vi "Set2DPlots.vi"(2 "error in (no error)":errorcluster, 3 "ScanCoords [mm]":T1, 4 "Order selection":u16(ring)=1 items=["X->Z->Y"=6, "Y->Z->X"=5, "Z->X->Y"=3, "Y->X->Z"=2, "Z->Y->X"=4, "X->Y->Z"=1], 5 "2D graph 3":refnum<vi>) -> (0 "error out":errorcluster, 1 "initialized array":dbl[][](array[numeric]))   [LabVIEW 2015]
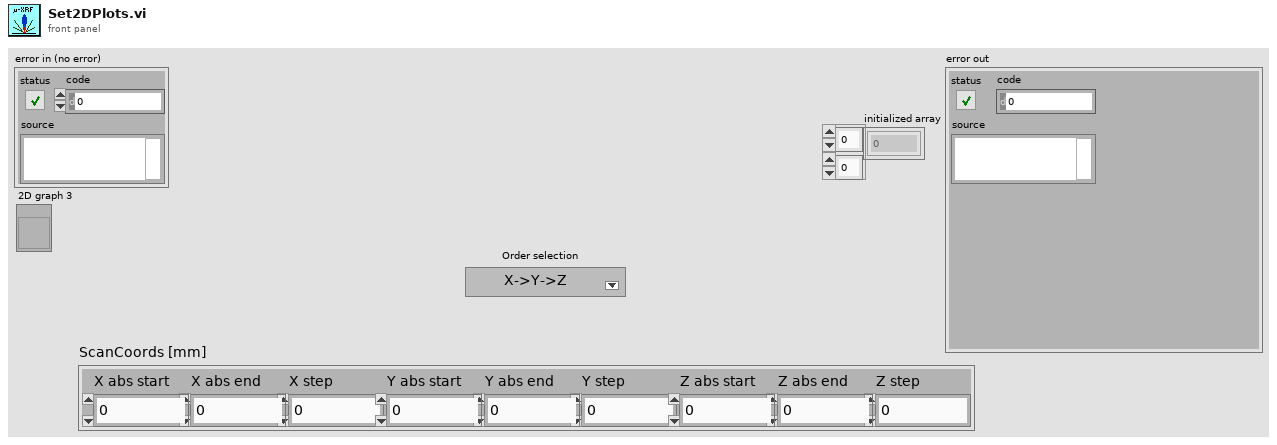
[diagram p1: front panel]
types:
  T1 = cluster{"X abs start":dbl, "X abs end":dbl, "Y abs start":dbl, "Y abs end":dbl, "Z abs start":dbl, "Z abs end":dbl, "X step":dbl, "Y step":dbl, "Z step":dbl}
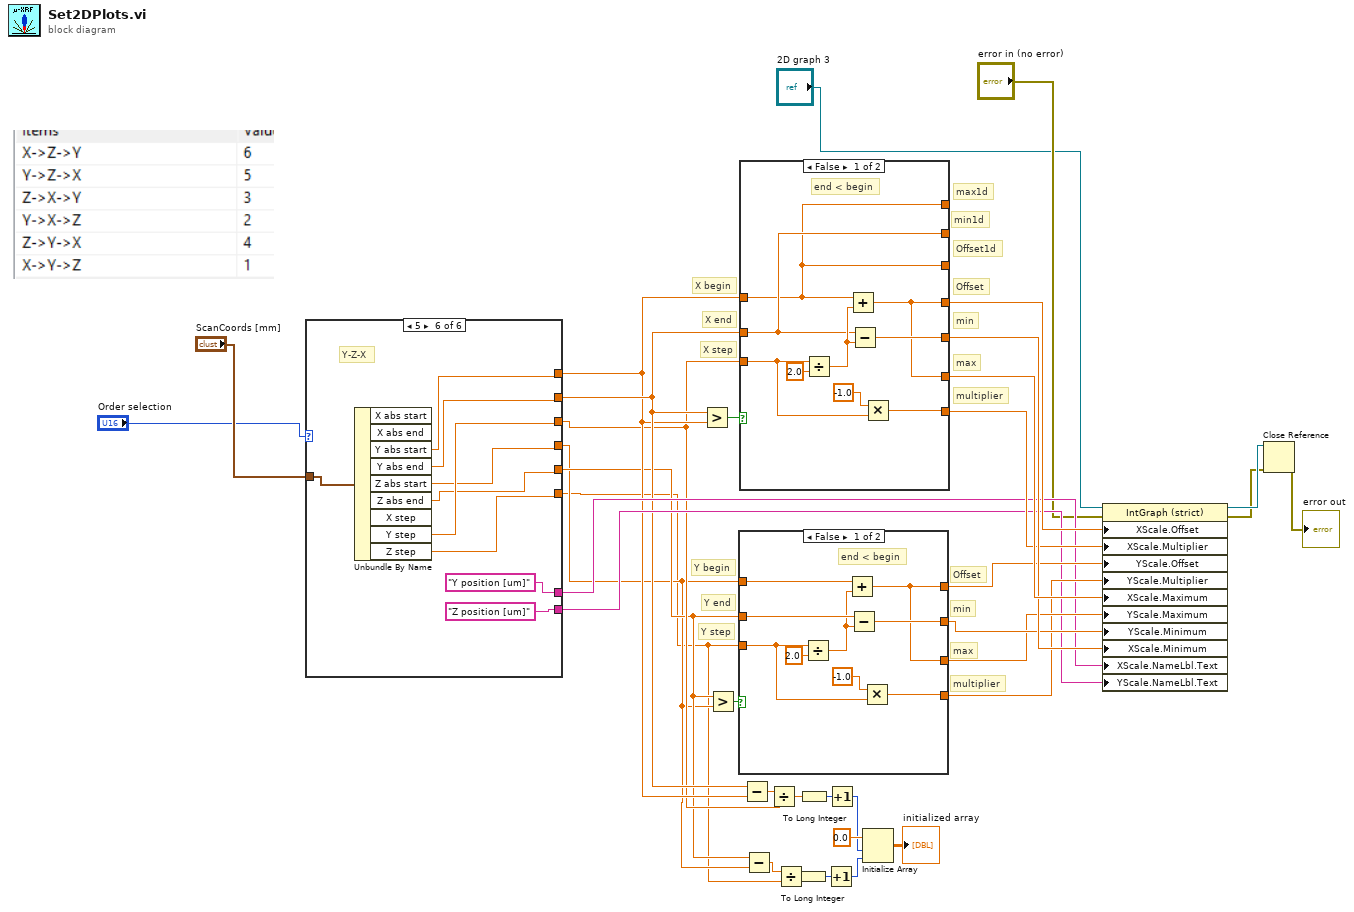
[diagram p0: block diagram]
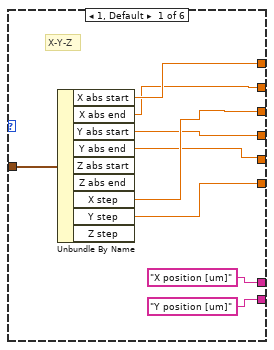
[diagram p2: hidden frame]
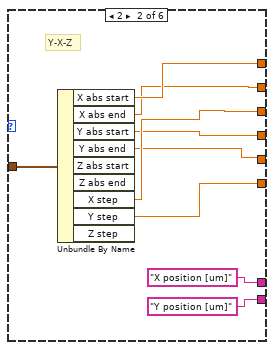
[diagram p3: hidden frame]
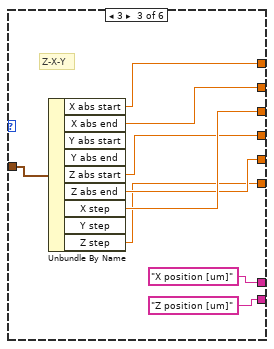
[diagram p4: hidden frame]
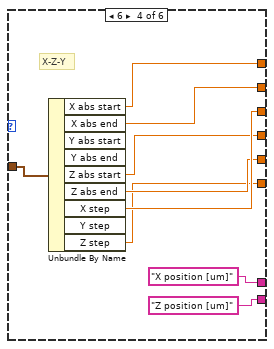
[diagram p5: hidden frame]
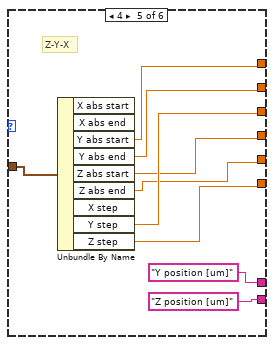
[diagram p6: hidden frame]
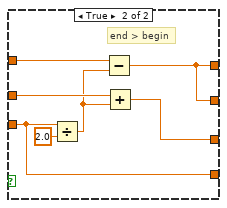
[diagram p7: hidden frame]
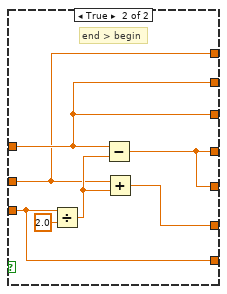
[diagram p8: hidden frame]
diagram:
  # "max1d"
  # "min1d"
  # "Offset1d"
  # "multiplier"
  # "min"
  # "max"
  # "Offset"
  # "Y step"
  # "Y end"
  # "Y begin"
  # "multiplier"
  # "min"
  # "max"
  # "Offset"
  # "X step"
  # "X end"
  # "X begin"
  n1 = case shown="5" "Order selection" {
    tunnel: [w40 w49 w58 w67 w76 w85] -> w12
    tunnel: [w41 w50 w59 w68 w77 w86] -> w11
    tunnel: [w36 w45 w55 w64 w73 w82] -> w9
    tunnel: [w37 w46 w56 w65 w74 w83] -> w8
    tunnel: [w39 w48 w57 w66 w75 w84] -> w10
    tunnel: [w38 w47 w54 w63 w72 w81] -> w7
    tunnel: ["X position [um]" "X position [um]" "X position [um]" "X position [um]" "Y position [um]" "Y position [um]"] -> w24
    tunnel: ["Y position [um]" "Y position [um]" "Z position [um]" "Z position [um]" "Z position [um]" "Z position [um]"] -> w23
    tunnel: "ScanCoords [mm]" -> [w42 w51 w60 w69 w78 w87]
    frame 1, Default {
      # "X-Y-Z"
      n2 = Unbundle By Name(w42) -> ("X abs start"=w41:dbl, "X abs end"=w40:dbl, "Y abs start"=w37:dbl, "Y abs end"=w36:dbl, "X step"=w39:dbl, "Y step"=w38:dbl)  [unwired: 3 out]
    }
    frame 2 {
      # "Y-X-Z"
      n3 = Unbundle By Name(w51) -> ("X abs start"=w50:dbl, "X abs end"=w49:dbl, "Y abs start"=w46:dbl, "Y abs end"=w45:dbl, "X step"=w48:dbl, "Y step"=w47:dbl)  [unwired: 3 out]
    }
    frame 3 {
      # "Z-X-Y"
      n4 = Unbundle By Name(w60) -> ("X abs start"=w59:dbl, "X abs end"=w58:dbl, "Z abs start"=w56:dbl, "Z abs end"=w55:dbl, "X step"=w57:dbl, "Z step"=w54:dbl)  [unwired: 3 out]
    }
    frame 6 {
      # "X-Z-Y"
      n5 = Unbundle By Name(w69) -> ("X abs start"=w68:dbl, "X abs end"=w67:dbl, "Z abs start"=w65:dbl, "Z abs end"=w64:dbl, "X step"=w66:dbl, "Z step"=w63:dbl)  [unwired: 3 out]
    }
    frame 4 {
      # "Z-Y-X"
      n6 = Unbundle By Name(w78) -> ("Y abs start"=w77:dbl, "Y abs end"=w76:dbl, "Z abs start"=w74:dbl, "Z abs end"=w73:dbl, "Y step"=w75:dbl, "Z step"=w72:dbl)  [unwired: 3 out]
    }
    frame 5 {
      # "Y-Z-X"
      n7 = Unbundle By Name(w87) -> ("Y abs start"=w86:dbl, "Y abs end"=w85:dbl, "Z abs start"=w83:dbl, "Z abs end"=w82:dbl, "Y step"=w84:dbl, "Z step"=w81:dbl)  [unwired: 3 out]
    }
  }
  n8 = Greater?(x=w12, y=w11) -> (0:w35:bool)
  n9 = Greater?(x=w9, y=w8) -> (0:w31:bool)
  n10 = case shown="False" w31 {
    tunnel: w8 -> [w94 w104]
    tunnel: w9 -> [w93 w103]
    tunnel: w7 -> [w96 w99]
    tunnel: [w90 w100] -> w27
    tunnel: [w90 w101] -> w29
    tunnel: [w91 w100] -> w30
    tunnel: [w95 w99] -> w28
    frame False {
      # "end < begin"
      n11 = Divide(x=w96, y=2.0) -> (x/y=w92:dbl)
      n12 = Add(x=w94, y=w92) -> (x+y=w90:dbl)
      n13 = Subtract(x=w93, y=w92) -> (x-y=w91:dbl)
      n14 = Multiply(x=-1.0 ("t"), y=w96) -> (x*y=w95:dbl)
    }
    frame True {
      # "end > begin"
      n15 = Divide(x=w99, y=2.0) -> (x/y=w102:dbl)
      n16 = Subtract(x=w104, y=w102) -> (x-y=w100:dbl)
      n17 = Add(x=w103, y=w102) -> (x+y=w101:dbl)
    }
  }
  n18 = case shown="False" w35 {
    tunnel: w11 -> [w106 w116]
    tunnel: w12 -> [w107 w115]
    tunnel: w10 -> [w112 w117]
    tunnel: [w108 w118] -> w34
    tunnel: [w108 w119] -> w33
    tunnel: [w109 w118] -> w32
    tunnel: [w111 w117] -> w26
    tunnel: [w106 w116] -> _
    tunnel: [w107 w116] -> _
    tunnel: [w106 w115] -> _
    frame False {
      # "end < begin"
      n19 = Divide(x=w112, y=2.0) -> (x/y=w110:dbl)
      n20 = Add(x=w106, y=w110) -> (x+y=w108:dbl)
      n21 = Subtract(x=w107, y=w110) -> (x-y=w109:dbl)
      n22 = Multiply(x=-1.0 ("t"), y=w112) -> (x*y=w111:dbl)
    }
    frame True {
      # "end > begin"
      n23 = Divide(x=w117, y=2.0) -> (x/y=w120:dbl)
      n24 = Subtract(x=w116, y=w120) -> (x-y=w118:dbl)
      n25 = Add(x=w115, y=w120) -> (x+y=w119:dbl)
    }
  }
  n26 = Subtract(x=w12, y=w11) -> (x-y=w20:dbl)
  n27 = Subtract(x=w9, y=w8) -> (x-y=w19:dbl)
  n28 = Divide(x=w20, y=w10) -> (x/y=w18:dbl)
  n29 = Divide(x=w19, y=w7) -> (x/y=w17:dbl)
  n30 = To Long Integer(number=w17) -> (32bit integer=w16:i32)
  n31 = To Long Integer(number=w18) -> (32bit integer=w14:i32)
  n32 = Increment(x=w16) -> (x+1=w15:i32)
  n33 = Increment(x=w14) -> (x+1=w13:i32)
  n34 = Initialize Array(0.0 ("element"), w13, w15) -> (→"initialized array":dbl[][])
  n35 = property class="IntGraph (strict)"(reference="2D graph 3", error in="error in (no error)", "XScale.Offset"=w34, "XScale.Multiplier"=w26, "YScale.Offset"=w27, "YScale.Multiplier"=w28, "XScale.Maximum"=w33, "YScale.Maximum"=w29, "YScale.Minimum"=w30, "XScale.Minimum"=w32, "XScale.NameLbl.Text"=w24, "YScale.NameLbl.Text"=w23) -> (reference out=w4:refnum<vi>, error out=w3:errorcluster)
  n36 = Close Reference(reference=w4, error in (no error)=w3) -> (error out=→"error out":errorcluster)
